vi "Test A.vi"(6 "Station":T1(ring), 8 "error in (no error)":errorcluster) -> (0 "error out":errorcluster)   [LabVIEW 2019, in "Sequence Example.lvlib"]
uses:
  Sequence Example.lvlib
  d31799f9-9e59-4a03-9ea0-60b3ce935fd9.vi
  ef1199a8-5428-4dd5-a187-ce5407e14e1f.vi
  <vilib>/Utility/Data Type/Get Type Information.vi
  Almost Equal.vi
  Unit Test Engine Tools.lvlib
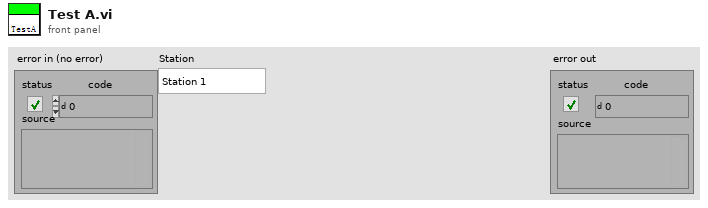
[diagram p1: front panel]
types:
  T1 = enum16{"Station 1", "Station 2", "Station 3", "Station 4"}
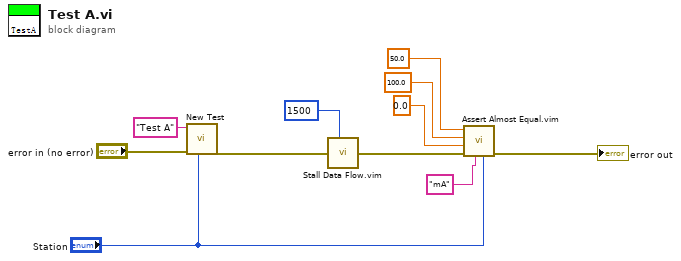
[diagram p0: block diagram]
diagram:
  n1 = call "New Test.vi"("Station"="Station", "error in (no error)"="error in (no error)", "Test"="Test A") -> ("error out"=w9:errorcluster)  [unwired: 8 in]
  n2 = call "Stall Data Flow.vim"("value in"=w9, "milliseconds to wait"=u32 1500) -> ("value out"=w7:errorcluster)  [unwired: 1 out]
  n3 = call "Assert Almost Equal.vim"("Station"="Station", "Unit"="mA", "error in (no error)"=w7, "Low limit"=0.0, "High limit"=100.0, "X"=50.0) -> ("error out"=→"error out":errorcluster)  [unwired: 5 in]
